vi "Rotation Control.vi"(0 "Feedback":dbl, 2 "Rotation Setpoints":T1, 3 "PID gains":T2={"Rotation_P_Gain"=0.02, "Rotation_I_Gain"=0.0, "Rotation_D_Gain"=0.0} {"Rotation_D_Gain" format="%.5f"; "Rotation_I_Gain" format="%.5f"; "Rotation_P_Gain" format="%.5f"}, 7 "Axis 2":dbl, 9 "RotationDesired":dbl) -> (14 "PID PWM 5 Output":dbl, 17 "AI 5 Setpoint (Volts)":dbl format="%.2f")   [LabVIEW 2011]
uses:
  Robot Global Data.vi
panel:
  in  "Down Rate":dbl=0.1
  in  "Rate":dbl=0.1
  # "dont change here, loaded globally"
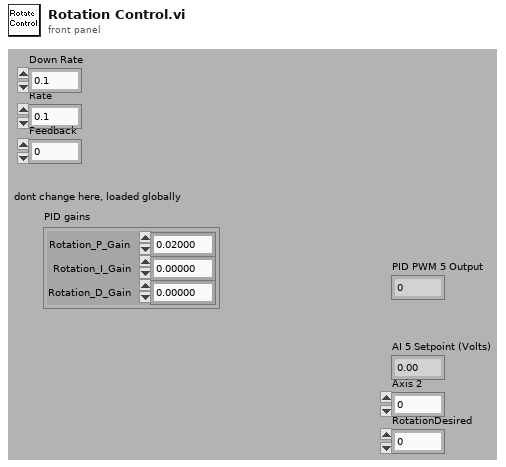
[diagram p1: front panel]
types:
  T1 = cluster{"Rotation Point F1":dbl, "Rotation Point F2":dbl, "Rotation Point F3":dbl, "Rotation Point F4":dbl, "Tube Carry":dbl, "Rotation Point B1":dbl, "Rotation Point B2":dbl, "Rotation Point B3":dbl, "Rotation Point B4":dbl, "Tube Carry Back":dbl}
  T2 = cluster{"Rotation_P_Gain":dbl, "Rotation_I_Gain":dbl, "Rotation_D_Gain":dbl}
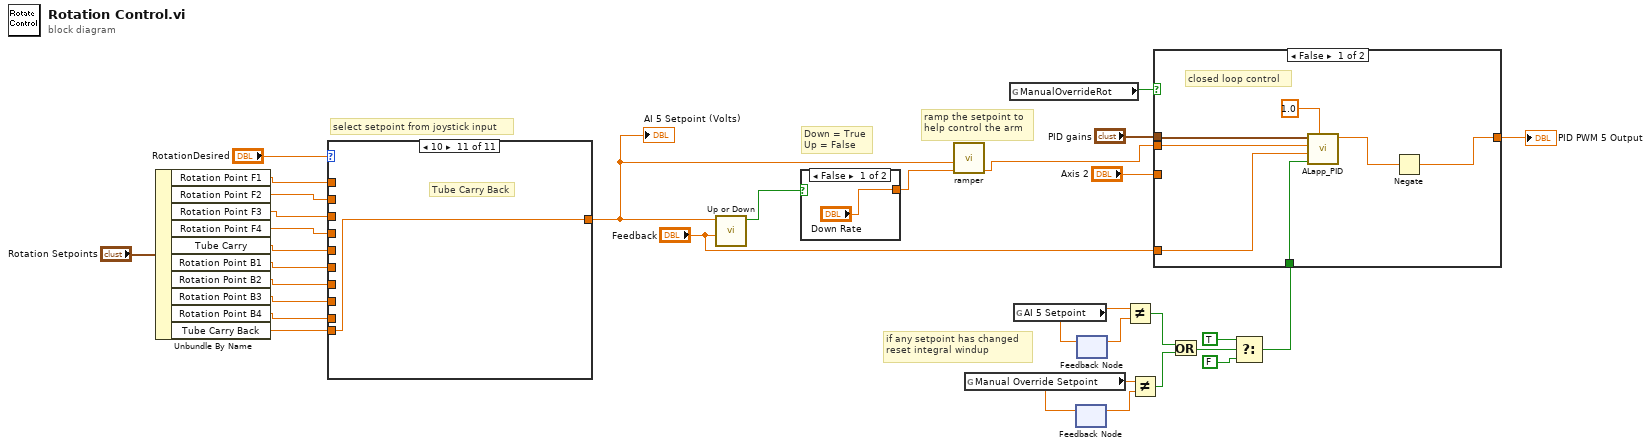
[diagram p0: block diagram]
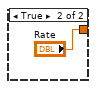
[diagram p2: hidden frame]
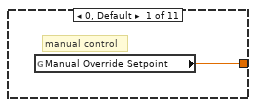
[diagram p3: hidden frame]
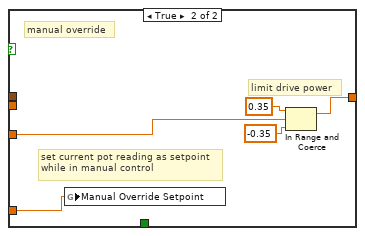
[diagram p13: hidden frame]
diagram:
  # "ramp the setpoint to\nhelp control the arm"
  # "select setpoint from joystick input"
  # "if any setpoint has changed\nreset integral windup"
  # "Down = True\nUp = False"
  n1 = Unbundle By Name("Rotation Setpoints") -> ("Rotation Point F1"=w31:dbl, "Rotation Point F2"=w30:dbl, "Rotation Point F3"=w29:dbl, "Rotation Point F4"=w28:dbl, "Tube Carry"=w27:dbl, "Rotation Point B1"=w26:dbl, "Rotation Point B2"=w25:dbl, "Rotation Point B3"=w24:dbl, "Rotation Point B4"=w23:dbl, "Tube Carry Back"=w18:dbl)
  n2 = case shown="10" "RotationDesired" {
    tunnel: [w32 w33 w34 w35 w36 w37 w38 w39 w40 w41 w42] -> w11
    tunnel: w31 -> [_ w33 _ _ _ _ _ _ _ _ _]
    tunnel: w30 -> [_ _ w34 _ _ _ _ _ _ _ _]
    tunnel: w29 -> [_ _ _ w35 _ _ _ _ _ _ _]
    tunnel: w28 -> [_ _ _ _ w36 _ _ _ _ _ _]
    tunnel: w27 -> [_ _ _ _ _ w37 _ _ _ _ _]
    tunnel: w26 -> [_ _ _ _ _ _ _ _ _ w41 _]
    tunnel: w25 -> [_ _ _ _ _ _ _ _ w40 _ _]
    tunnel: w24 -> [_ _ _ _ _ _ _ w39 _ _ _]
    tunnel: w23 -> [_ _ _ _ _ _ w38 _ _ _ _]
    tunnel: w18 -> [_ _ _ _ _ _ _ _ _ _ w42]
    frame 0, Default {
      # "manual control"
      n3 = global read "Robot Global Data.vi" "Manual Override Setpoint"() -> (w32:dbl)
    }
    frame 1 {
      # "pick up front"
    }
    frame 2 {
      # "low rack"
    }
    frame 3 {
      # "mid rack"
    }
    frame 4 {
      # "high rack"
    }
    frame 5 {
      # "neutral (tube carry)"
    }
    frame 6 {
      # "pick up (back)"
    }
    frame 7 {
      # "low rack (back)"
    }
    frame 8 {
      # "mid rack (back)"
    }
    frame 9 {
      # "high rack (back)"
    }
    frame 10 {
      # "Tube Carry Back"
    }
  }
  "AI 5 Setpoint (Volts)" <- w11
  n4 = call "Up or Down.vi"("Current Position (deg)"="Feedback", "Current Setpoint (deg)"=w11) -> ("Moving UP?"=w8:bool)  [unwired: 9 out]
  n5 = case shown="False" w8 {
    tunnel: ["Down Rate" "Rate"] -> w4
    frame False {
    }
    frame True {
    }
  }
  n6 = call "ramper.vi"("Rate"=w4, "Target Setpoint"=w11) -> ("Current Setpoint"=w1:dbl)  [unwired: 2 in, 7 out]
  n7 = global read "Robot Global Data.vi" "Manual Override Setpoint"() -> (w15:dbl)
  n8 = global read "Robot Global Data.vi" "ManualOverrideRot"() -> (w5:bool)
  n9 = global read "Robot Global Data.vi" "AI 5 Setpoint"() -> (w17:dbl)
  n10 = feedback-in #1(w15) -> ()
  n11 = feedback #1() -> (w14:dbl)  [unwired: 1 out]
  n12 = feedback-in #2(w17) -> ()
  n13 = feedback #2() -> (w21:dbl)  [unwired: 1 out]
  n14 = Not Equal?(x=w17, y=w21) -> (x != y?=w12:bool)
  n15 = Not Equal?(x=w15, y=w14) -> (x != y?=w13:bool)
  n16 = Or(x=w12, y=w13) -> (x .or. y?=w9:bool)
  n17 = Select(t=TRUE ("AI 5 Rotation Complete"), s=w9, f=FALSE ("AI 5 Rotation Complete")) -> (s? t:f=w3:bool)
  n18 = case shown="False" w5 {
    tunnel: [w45 w55] -> w7
    tunnel: w1 -> [w49 _]
    tunnel: "Feedback" -> [w48 w56]
    tunnel: w3 -> [w51 _]
    tunnel: "PID gains" -> [w50 _]
    tunnel: "Axis 2" -> [_ w54]
    frame False {
      # "closed loop control"
      n19 = call "ALapp_PID.vi"(0:w50, "Setpoint"=w49, "Feedback"=w48, "integral reset"=w51, "PID Out Max"=1.0) -> ("Motor Output"=w46:dbl)  [unwired: 1 in, 4 out]
      n20 = Negate(x=w46) -> (-x=w45:dbl)
    }
    frame True {
      # "limit drive power"
      # "manual override"
      # "set current pot reading as setpoint\nwhile in manual control"
      n21 = global write "Robot Global Data.vi" "Manual Override Setpoint"(w56) -> ()
      n22 = In Range and Coerce(upper limit=0.35, x=w54, lower limit=-0.35) -> (coerced(x)=w55:dbl)  [unwired: 1 out]
    }
  }
  "PID PWM 5 Output" <- w7
